vi "FT-IR EVID-Codes External Data.vi"(0 "Startadresse":i32, 1 "Smoothing?":bool, 5 "Anzahl":i32, 7 "Rolling Average Settings":T1={"Average"=1, "Average via AK:"=FALSE, "Average IAG Software:"=FALSE} {"Average" min=1 max=600}, 9 "1Hz/5Hz Leitsystem":T2=1 items=["1Hz"=1, "5Hz"=5, "10Hz"=10], 11 "1Hz/5Hz Gerät":T2=1 items=["1Hz"=1, "5Hz"=5, "10Hz"=10], 12 "Aktionen":T3) -> (4 "Startadresse":i32, 6 "Anzahl":i32, 8 "Rolling Average Settings":T1={"Average"=1, "Average via AK:"=FALSE, "Average IAG Software:"=FALSE} {"Average" min=1 max=600}, 10 "1Hz/5Hz Leitsystem":T2=1 items=["1Hz"=1, "5Hz"=5, "10Hz"=10], 14 "Smoothing?":bool, 15 "1Hz/5Hz Gerät":T2=1 items=["1Hz"=1, "5Hz"=5, "10Hz"=10])   [LabVIEW 2020, in "FT-IR.lvlib"]
uses:
  FT-IR.lvlib
  Aktionen EVID-Codes.ctl
  1Hz-5Hz Geraet.ctl
  Rolling Average Settings.ctl
  <vilib>/Utility/config.llb/Read Key (I32).vi
  <vilib>/Utility/config.llb/Read Key (Boolean).vi
  <vilib>/Utility/config.llb/Read Key (U32).vi
  <vilib>/Utility/config.llb/Write Key (I32).vi
  <vilib>/Utility/config.llb/Write Key (Boolean).vi
  <vilib>/Utility/config.llb/Write Key (U32).vi
  <vilib>/Utility/config.llb/NI_LVConfig.lvlib
  Allgemein/allgemeine Sub-VIs.lvlib
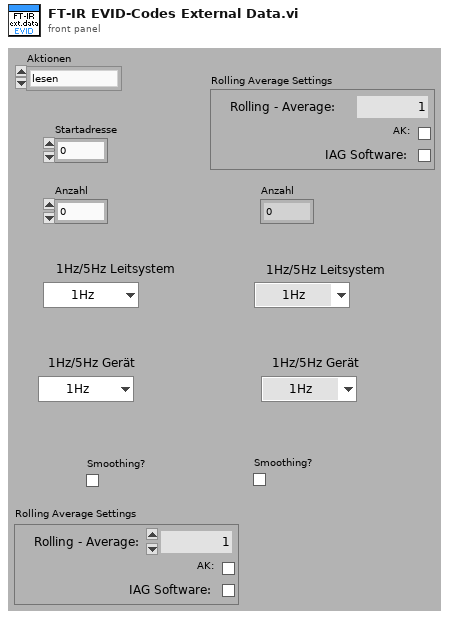
[diagram p1: front panel]
types:
  T1 = typedef "FT-IR.lvlib/Rolling Average Settings.ctl" = cluster{"Average":u32, "Average via AK:":bool, "Average IAG Software:":bool}
  T2 = typedef "FT-IR.lvlib/1Hz-5Hz Geraet.ctl" = u16
  T3 = typedef "FT-IR.lvlib/Aktionen EVID-Codes.ctl" = enum16{"lesen", "setzen", "laden", "speichern", "1Hz/5Hz", "Smoothing", "Rolling Average"}
  T4 = typedef "NI_LVConfig.lvlib/Config Data RefNum.ctl" = refnum<k1>
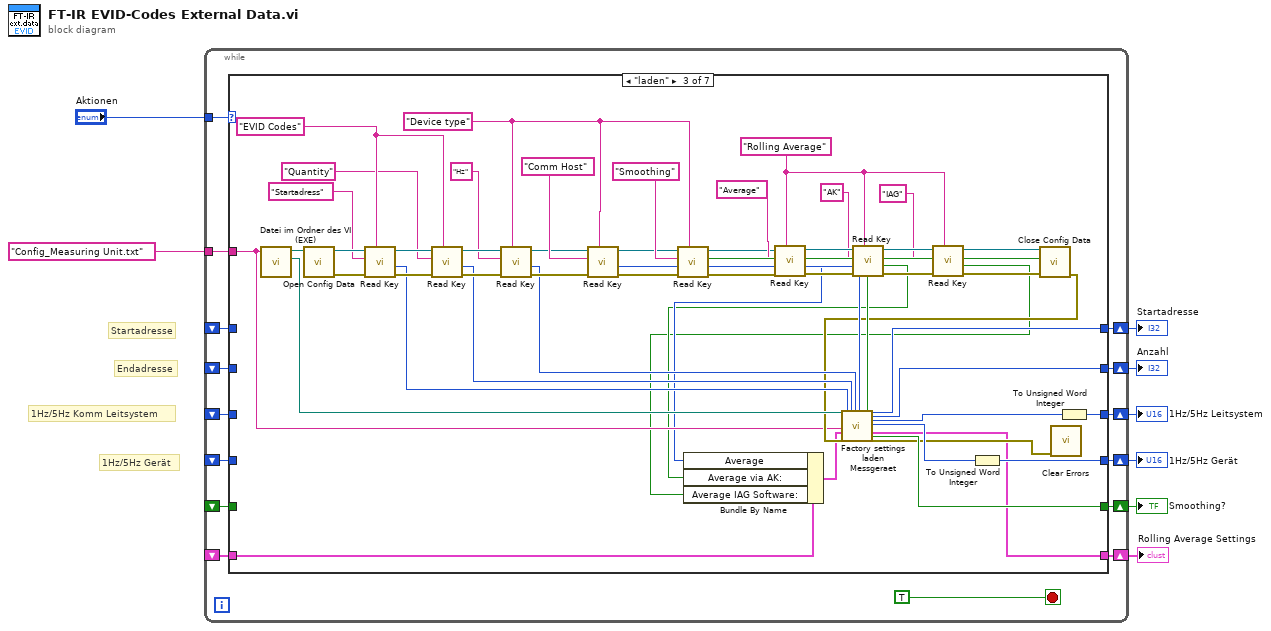
[diagram p0: block diagram]
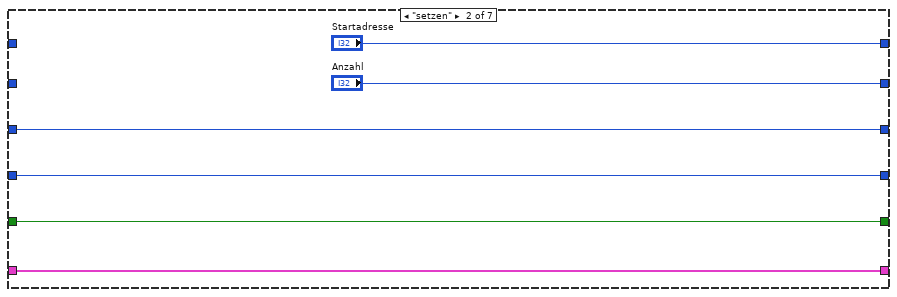
[diagram p3: hidden frame]
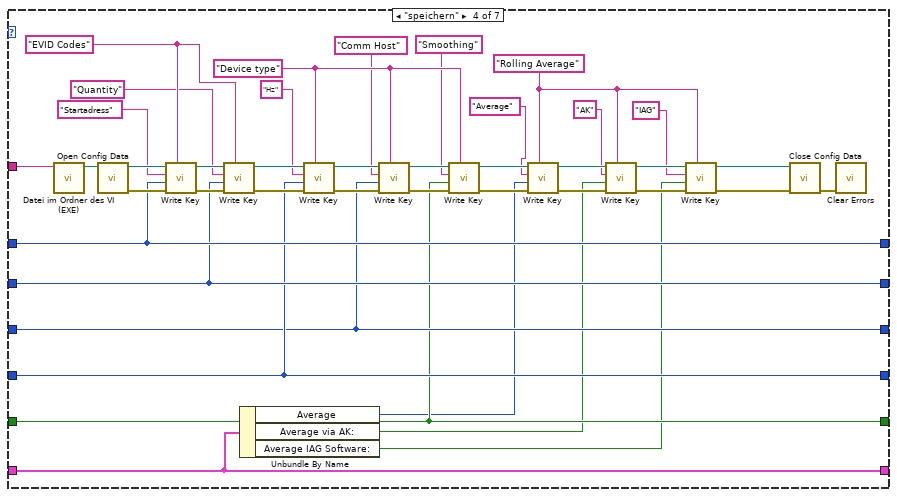
[diagram p4: hidden frame]
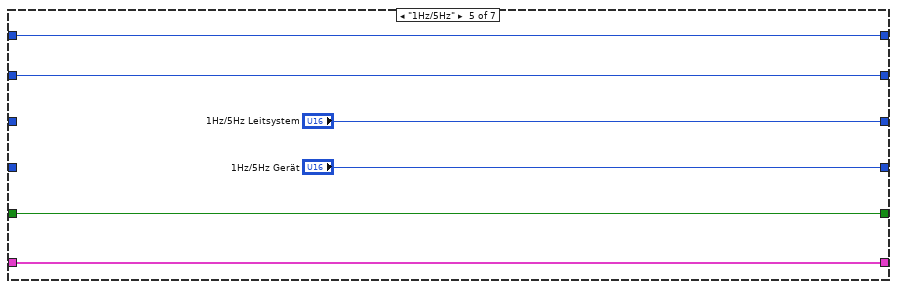
[diagram p5: hidden frame]
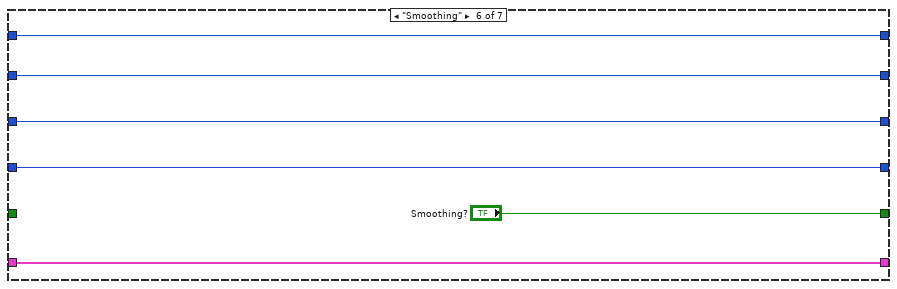
[diagram p6: hidden frame]
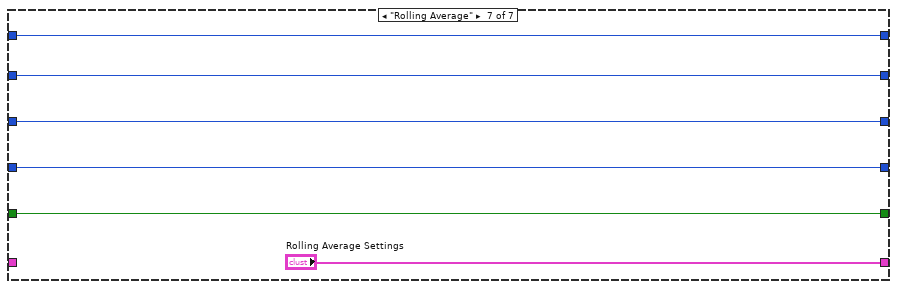
[diagram p7: hidden frame]
diagram:
  # "1Hz/5Hz Komm Leitsystem"
  # "1Hz/5Hz Gerät"
  # "Endadresse"
  # "Startadresse"
  n1 = while {
    tunnel: "Aktionen" -> [w23]
    shift-right: [w21] -> w7
    shift-left: _ -> [w19]
    shift-right: [w20] -> w6
    shift-left: _ -> [w18]
    shift-right: [w17] -> w5
    shift-left: _ -> [w16]
    shift-right: [w14] -> w4
    shift-left: _ -> [w15]
    shift-right: [w12] -> w3
    shift-left: _ -> [w13]
    tunnel: "Config_Measuring Unit.txt" ("Dateiname") -> [w11]
    shift-right: [w10] -> w1
    shift-left: _ -> [w9]
    stop <- TRUE stop-if-true
    n2 = case shown="\"laden\"" w23 {
      tunnel: [w29 "Startadresse" w66 w121 w133 w138 w144] -> w21
      tunnel: [w28 "Anzahl" w64 w120 w134 w139 w145] -> w20
      tunnel: w19 -> [w29 _ _ w121 w133 w138 w144]
      tunnel: w18 -> [w28 _ _ w120 w134 w139 w145]
      tunnel: [w27 w33 w77 w115 "1Hz/5Hz Gerät" w141 w147] -> w17
      tunnel: w16 -> [w27 w33 _ w115 _ w141 w147]
      tunnel: w15 -> [w26 w32 _ w112 _ w140 w146]
      tunnel: [w26 w32 w73 w112 "1Hz/5Hz Leitsystem" w140 w146] -> w14
      tunnel: w13 -> [w25 w31 _ w109 w131 _ w143]
      tunnel: [w25 w31 w61 w109 w131 "Smoothing?" w143] -> w12
      tunnel: w11 -> [_ _ w54 w105 _ _ _]
      tunnel: [w24 w30 w53 w102 w130 w136 "Rolling Average Settings"] -> w10
      tunnel: w9 -> [w24 w30 w40 w102 w130 w136 _]
      frame "lesen", Default {
      }
      frame "setzen" {
      }
      frame "laden" {
        w48 = "Rolling Average" ("section")
        w68 = "Device type" ("section")
        w83 = "EVID Codes" ("section")
        n3 = call "Datei im Ordner des VI (EXE).vi"("Dateiname"=w54) -> ("Ordner des Haupt-VIs"=w57:path, "Dateipfad im Ordner des Haupt-VIs"=w88:path)  [unwired: 8 in, 1 out]
        n4 = call <vilib>:"Open Config Data.vi"("configuration file path"=w88) -> ("error out"=w85:errorcluster, "refnum"=w86:T4)  [unwired: 8 in, 1 out]
        n5 = call-poly <vilib>:"Read Key.vi"("section"=w83, "error in (no error)"=w85, "key"="Startadress", "refnum"=w86) -> ("error out"=w87:errorcluster, "value"=w67:i32, "refnum out"=w84:T4)  [unwired: 4 in, 1 out]
        n6 = call-poly <vilib>:"Read Key.vi"("section"=w83, "error in (no error)"=w87, "key"="Quantity", "refnum"=w84) -> ("error out"=w79:errorcluster, "value"=w65:i32, "refnum out"=w80:T4)  [unwired: 4 in, 1 out]
        n7 = call-poly <vilib>:"Read Key.vi"("section"=w68, "error in (no error)"=w79, "key"="Hz", "refnum"=w80) -> ("error out"=w74:errorcluster, "value"=w60:i32, "refnum out"=w75:T4)  [unwired: 4 in, 1 out]
        n8 = call-poly <vilib>:"Read Key.vi"("section"=w68, "error in (no error)"=w74, "key"="Comm Host", "refnum"=w75) -> ("error out"=w69:errorcluster, "value"=w59:i32, "refnum out"=w70:T4)  [unwired: 4 in, 1 out]
        n9 = call-poly <vilib>:"Read Key.vi"("section"=w68, "error in (no error)"=w69, "key"="Smoothing", "refnum"=w70) -> ("error out"=w41:errorcluster, "value"=w58:bool, "found?"=w71:bool, "refnum out"=w42:T4)  [unwired: 4 in]
        n10 = call-poly <vilib>:"Read Key.vi"("section"=w48, "error in (no error)"=w41, "key"="Average" ("section"), "refnum"=w42) -> ("error out"=w52:errorcluster, "value"=w38:u32, "refnum out"=w51:T4)  [unwired: 4 in, 1 out]
        n11 = call-poly <vilib>:"Read Key.vi"("section"=w48, "error in (no error)"=w52, "key"="AK" ("section"), "refnum"=w51) -> ("error out"=w50:errorcluster, "value"=w37:bool, "refnum out"=w49:T4)  [unwired: 4 in, 1 out]
        n12 = call-poly <vilib>:"Read Key.vi"("section"=w48, "error in (no error)"=w50, "key"="IAG" ("section"), "refnum"=w49) -> ("error out"=w44:errorcluster, "value"=w36:bool, "refnum out"=w43:T4)  [unwired: 4 in, 1 out]
        n13 = Bundle By Name(cluster=w40, "Average"=w38, "Average via AK:"=w37, "Average IAG Software:"=w36) -> (w39:T1)
        n14 = call <vilib>:"Close Config Data.vi"("error in (no error)"=w44, "write file if changed (T)"=w71, "refnum"=w43) -> ("error out"=w56:errorcluster)  [unwired: 7 in, 1 out]
        n15 = call "Factory settings laden Messgeraet.vi"("Ordner des Haupt-VIs"=w57, "Dateiname"=w54, "Rolling Average Settings"=w39, "error in (no error)"=w56, "Startadresse"=w67, "Anzahl"=w65, "1Hz/5Hz Gerät"=w60, "1Hz/5Hz Leitsystem"=w59, "Smoothing?"=w58) -> ("Startadresse"=w66:i32, "Anzahl"=w64:i32, "1Hz/5Hz Leitsystem"=w63:T2, "1Hz/5Hz Gerät"=w62:T2, "Rolling Average Settings"=w53:T1, "Smoothing?"=w61:bool, "error out"=w55:errorcluster)  [unwired: 12 in]
        n16 = To Unsigned Word Integer(number=w62) -> (unsigned 16bit integer=w77:T2)
        n17 = call <vilib>:"Clear Errors.vi"("error in (no error)"=w55) -> ()  [unwired: 5 in, 2 out]
        n18 = To Unsigned Word Integer(number=w63) -> (unsigned 16bit integer=w73:T2)
      }
      frame "speichern" {
        w95 = "Rolling Average" ("section")
        w108 = "Device type" ("section")
        w124 = "EVID Codes" ("section")
        n19 = call "Datei im Ordner des VI (EXE).vi"("Dateiname"=w105) -> ("Dateipfad im Ordner des Haupt-VIs"=w129:path)  [unwired: 8 in, 2 out]
        n20 = call <vilib>:"Open Config Data.vi"("configuration file path"=w129) -> ("error out"=w126:errorcluster, "refnum"=w127:T4)  [unwired: 8 in, 1 out]
        n21 = call-poly <vilib>:"Write Key.vi"("section"=w124, "error in (no error)"=w126, "value"=w121, "key"="Startadress", "refnum"=w127) -> ("error out"=w128:errorcluster, "refnum out"=w125:T4)  [unwired: 4 in, 1 out]
        n22 = call-poly <vilib>:"Write Key.vi"("section"=w124, "error in (no error)"=w128, "value"=w120, "key"="Quantity", "refnum"=w125) -> ("error out"=w118:errorcluster, "refnum out"=w119:T4)  [unwired: 4 in, 1 out]
        n23 = Unbundle By Name(w102) -> ("Average"=w101:u32, "Average via AK:"=w91:bool, "Average IAG Software:"=w90:bool)
        n24 = call-poly <vilib>:"Write Key.vi"("section"=w108, "error in (no error)"=w118, "value"=w115, "key"="Hz", "refnum"=w119) -> ("error out"=w113:errorcluster, "refnum out"=w114:T4)  [unwired: 4 in, 1 out]
        n25 = call-poly <vilib>:"Write Key.vi"("section"=w108, "error in (no error)"=w113, "value"=w112, "key"="Comm Host" ("section"), "refnum"=w114) -> ("error out"=w110:errorcluster, "refnum out"=w111:T4)  [unwired: 4 in, 1 out]
        n26 = call-poly <vilib>:"Write Key.vi"("section"=w108, "error in (no error)"=w110, "value"=w109, "key"="Smoothing", "refnum"=w111) -> ("error out"=w103:errorcluster, "refnum out"=w104:T4)  [unwired: 4 in, 1 out]
        n27 = call-poly <vilib>:"Write Key.vi"("section"=w95, "error in (no error)"=w103, "value"=w101, "key"="Average" ("section"), "refnum"=w104) -> ("error out"=w100:errorcluster, "refnum out"=w99:T4)  [unwired: 4 in, 1 out]
        n28 = call-poly <vilib>:"Write Key.vi"("section"=w95, "error in (no error)"=w100, "value"=w91, "key"="AK" ("section"), "refnum"=w99) -> ("error out"=w98:errorcluster, "refnum out"=w96:T4)  [unwired: 4 in, 1 out]
        n29 = call-poly <vilib>:"Write Key.vi"("section"=w95, "error in (no error)"=w98, "value"=w90, "key"="IAG" ("section"), "refnum"=w96) -> ("error out"=w97:errorcluster, "refnum out"=w89:T4)  [unwired: 4 in, 1 out]
        n30 = call <vilib>:"Close Config Data.vi"("error in (no error)"=w97, "refnum"=w89) -> ("error out"=w117:errorcluster)  [unwired: 8 in, 1 out]
        n31 = call <vilib>:"Clear Errors.vi"("error in (no error)"=w117) -> ()  [unwired: 5 in, 2 out]
      }
      frame "1Hz/5Hz" {
      }
      frame "Smoothing" {
      }
      frame "Rolling Average" {
      }
    }
  }
  "Startadresse" <- w7
  "Anzahl" <- w6
  "1Hz/5Hz Gerät" <- w5
  "1Hz/5Hz Leitsystem" <- w4
  "Smoothing?" <- w3
  "Rolling Average Settings" <- w1
